vi "TeleopDriveFrwdsub.vi"(8 "SCALE":dbl=0.5 format="%#_13g", 9 "B VALUE":dbl=0.15 format="%#_13g", 10 "Deadband X value":dbl, 11 "Drive":dbl) -> (3 "Drive Output":dbl)   [LabVIEW 2017]
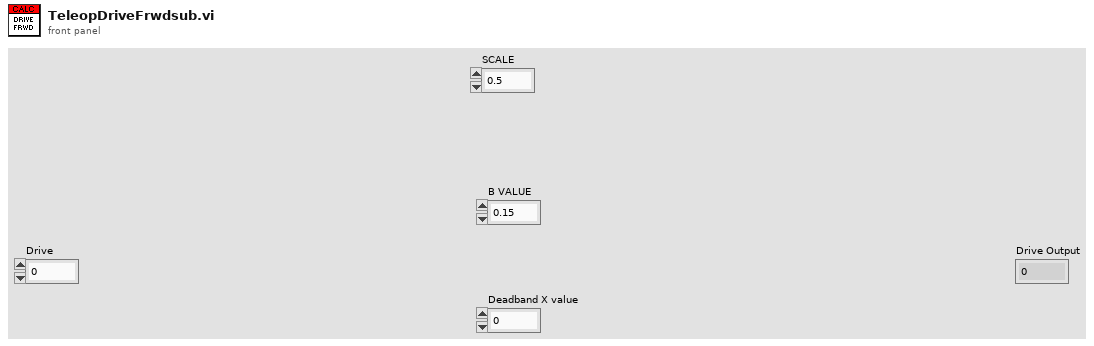
[diagram p1: front panel]
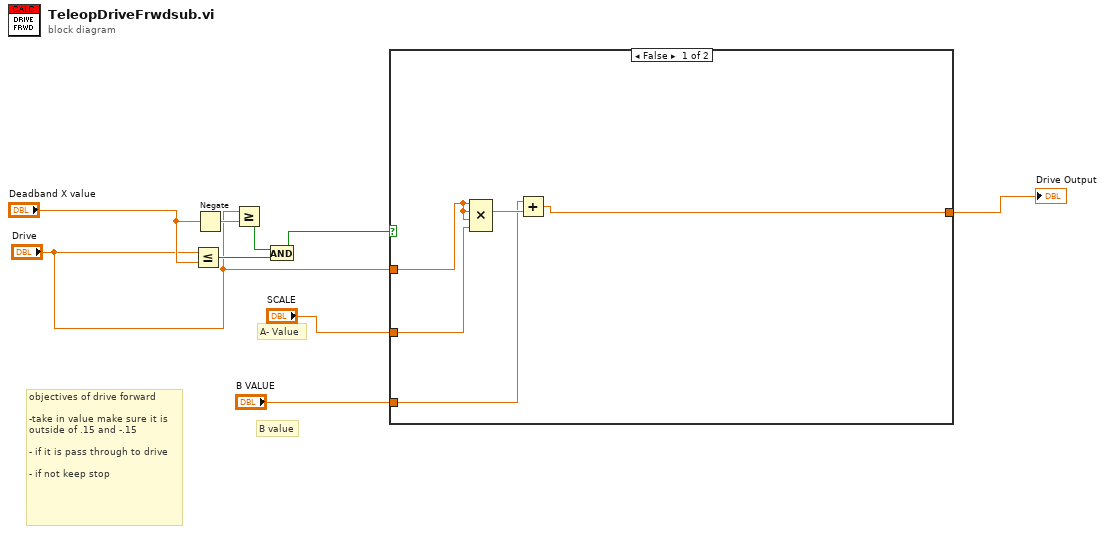
[diagram p0: block diagram]
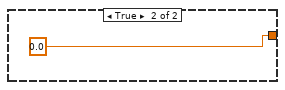
[diagram p2: hidden frame]
diagram:
  # "B value"
  # "A- Value"
  # "objectives of drive forward\n\n-take in value make sure it is \noutside of .15 and -.15\n\n- if it is pass through to drive\n\n- if not keep stop"
  n1 = Less Or Equal?(x="Drive", y="Deadband X value") -> (x <= y?=w7:bool)
  n2 = Negate(x="Deadband X value") -> (-x=w9:dbl)
  n3 = Greater Or Equal?(x="Drive", y=w9) -> (x >= y?=w6:bool)
  n4 = And(x=w6, y=w7) -> (x .and. y?=w5:bool)
  n5 = case shown="False" w5 {
    tunnel: "Drive" -> [w13 _]
    tunnel: [w12 0.0 ("Y axis value")] -> w3
    tunnel: "SCALE" -> [w11 _]
    tunnel: "B VALUE" -> [w10 _]
    frame False {
      n6 = Compound Arithmetic op=MULTIPLY(w13, w13, w13, w11) -> (w14:dbl)
      n7 = Add(x=w10, y=w14) -> (x+y=w12:dbl)
    }
    frame True {
    }
  }
  "Drive Output" <- w3
